vi "Auto Further Scale.vi"(10 "Time to wait (min 50ms)":dbl=100.0, 11 "Right?":bool=TRUE) -> ()   [LabVIEW 2017]
uses:
  LabVIEW_is_Under_Control.lib/Util/Unpack Gamepad/Button Cluster.ctl
  LabVIEW_is_Under_Control.lib/Util/Unpack Gamepad/D-Pad.ctl
  Team Code/Robot Global Data.vi
panel:
  out "Auto State":T1(ring)=enum."Finalizando"
  in  "Time_Limit_ Turn_2":dbl=1500.0 format="%#_13g"
  in  "Time_Limit_fwd_2":dbl=4500.0 format="%#_13g"
  in  "Time_Limit_Turn":dbl=2500.0 format="%#_13g"
  in  "Time_Limit_fwd":dbl=4000.0 format="%#_13g"
  in  "Time_Limit_fwd_3":dbl=2000.0 format="%#_13g"
  in  "Time to wait 3(min 50ms)":dbl=50.0
  in  "Delay Fwd 3":i32=100
  in  "DistanceScale":dbl=75.0
  in  "Delay Turn 2":i32=200
  in  "Turn 2":dbl=90.0 format="%#_13g"
  in  "Delay Fwd 2":i32=500
  in  "DistanceAfterTurn":dbl=450.0
  in  "Delay Turn":i32=600
  in  "Turn":dbl=-85.0 format="%#_13g"
  in  "Delay Fwd":i32=500
  in  "DistanceFwd":dbl=545.0
  in  "Time to wait 3 (min 50ms)":dbl=50.0
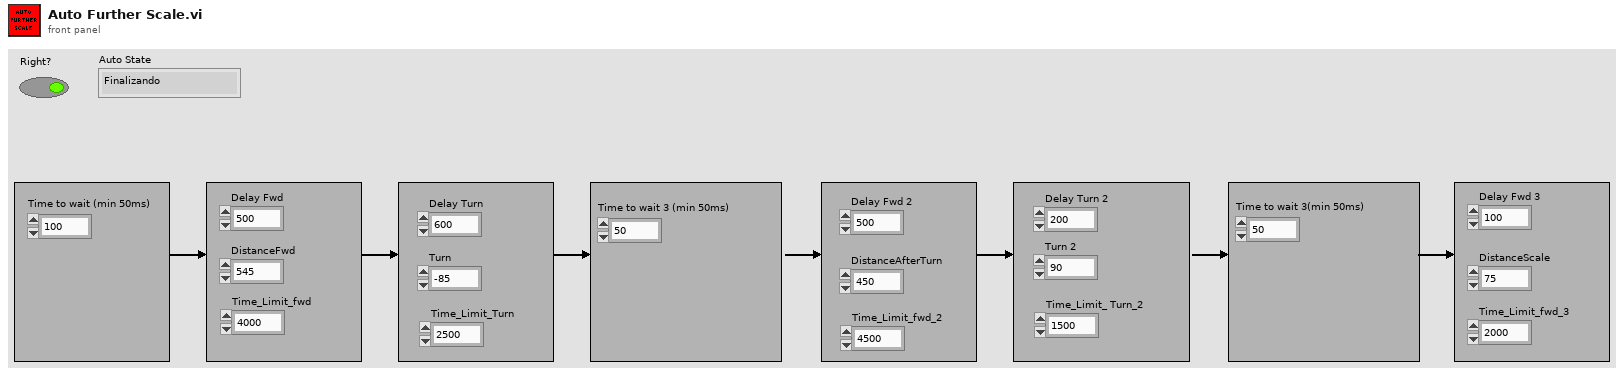
[diagram p1: front panel]
types:
  T1 = enum16{"Zerandosensor", "Andando", "Girando", "Zerandosensor2", "Andando2", "Girando2", "Zerandosensor3", "Andando3", "Score", "Finalizando", "Jogando"}
  T2 = enum16{"Zerandosensor", "Andando", "Girando", "Zerandosensor2", "Andando2", "Girando2", "Zerandosensor3", "Andando3", "Score", "Finalizando"}
  T3 = typedef "Button Cluster.ctl" = cluster{"Buttons[0]":bool, "Buttons[1]":bool, "Buttons[2]":bool, "Buttons[3]":bool, "Buttons[4]":bool, "Buttons[5]":bool, "Buttons[6]":bool, "Buttons[7]":bool, "Buttons[8]":bool, "Buttons[9]":bool}
  T4 = cluster{"proportional gain (Kc)":dbl, "integral time (Ti, min)":dbl, "derivative time (Td, min)":dbl}
  T5 = typedef "D-Pad.ctl" = cluster{"Top":bool, "Bottom":bool, "None":bool, "Right":bool, "Left":bool}
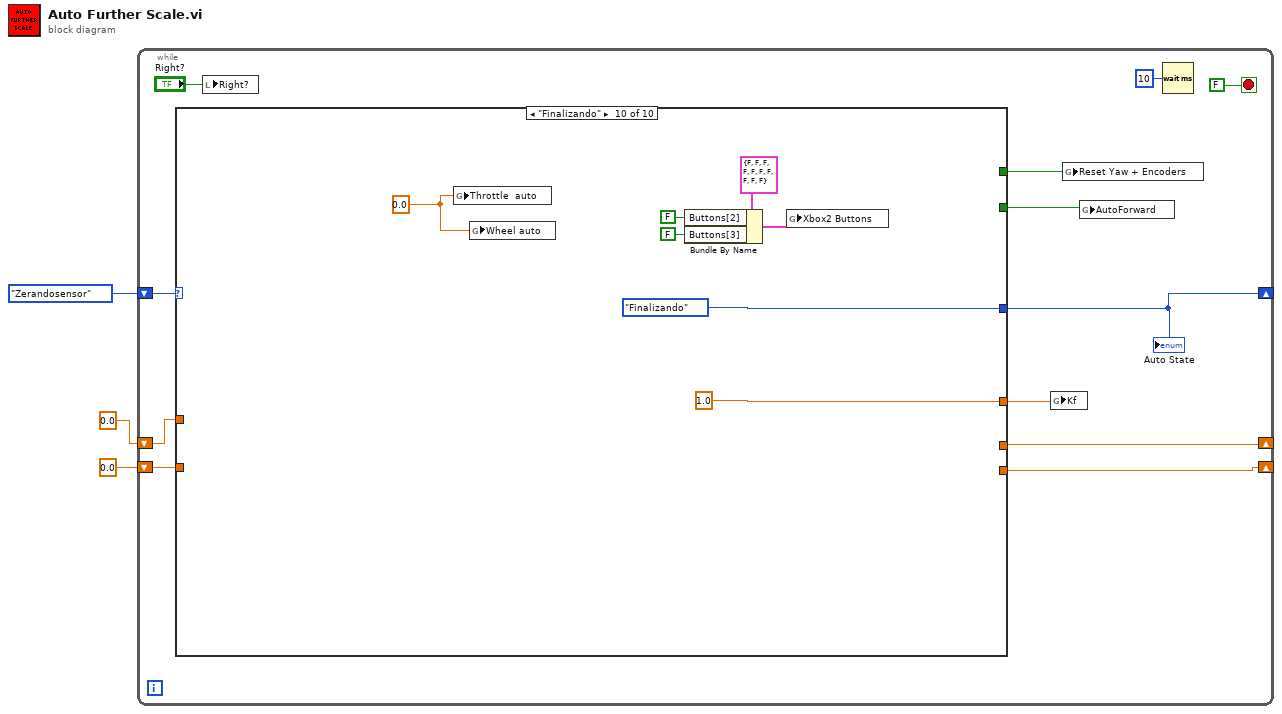
[diagram p0: block diagram]
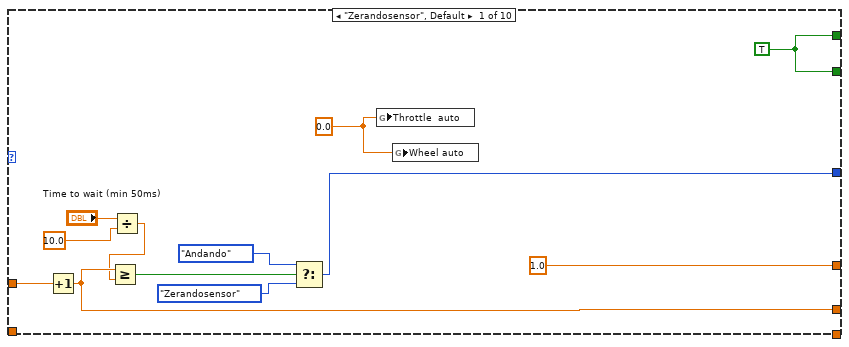
[diagram p2: hidden frame]
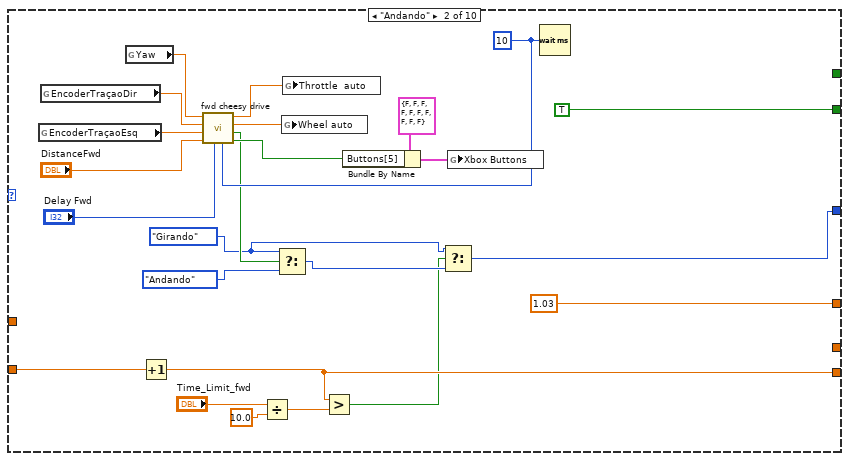
[diagram p3: hidden frame]
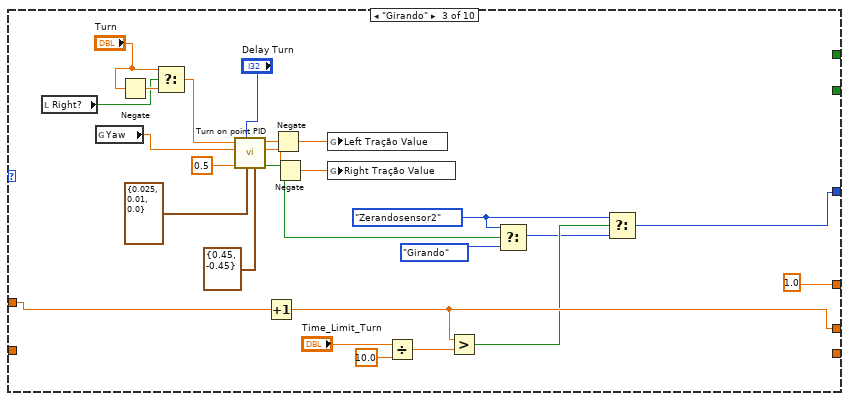
[diagram p4: hidden frame]
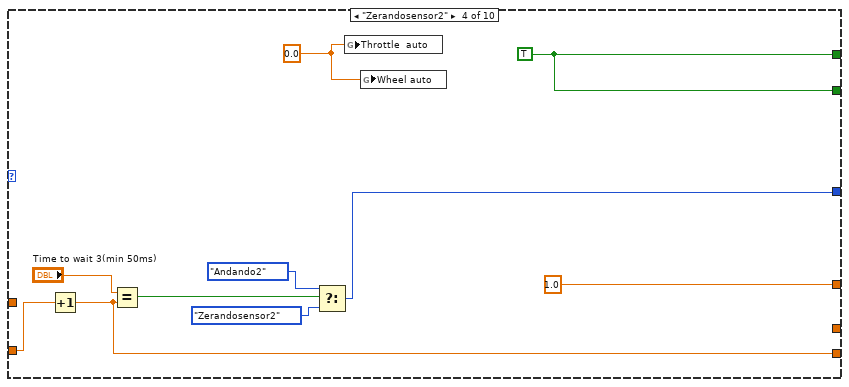
[diagram p5: hidden frame]
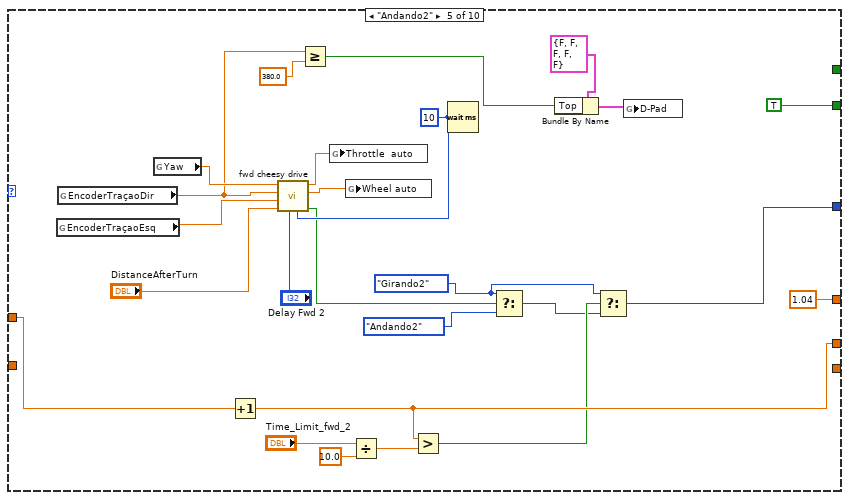
[diagram p6: hidden frame]
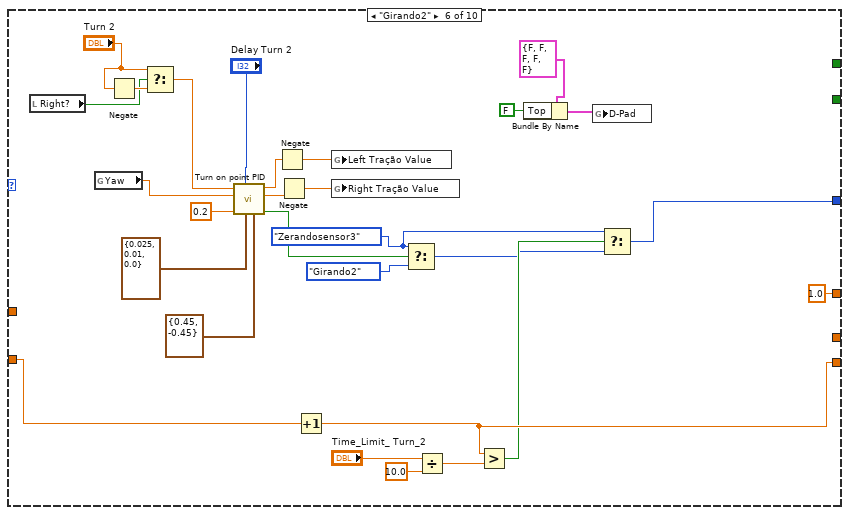
[diagram p7: hidden frame]
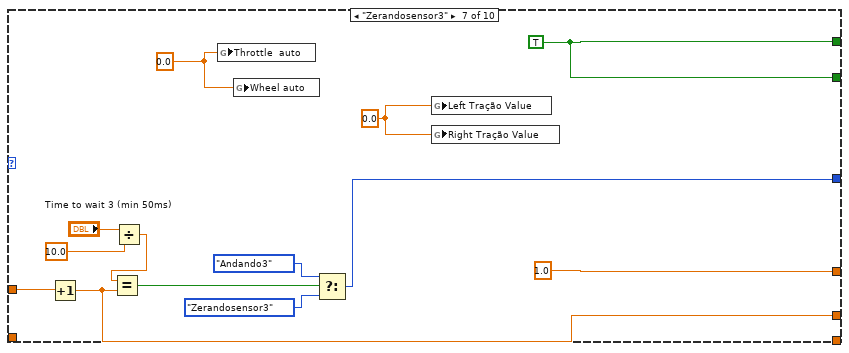
[diagram p8: hidden frame]
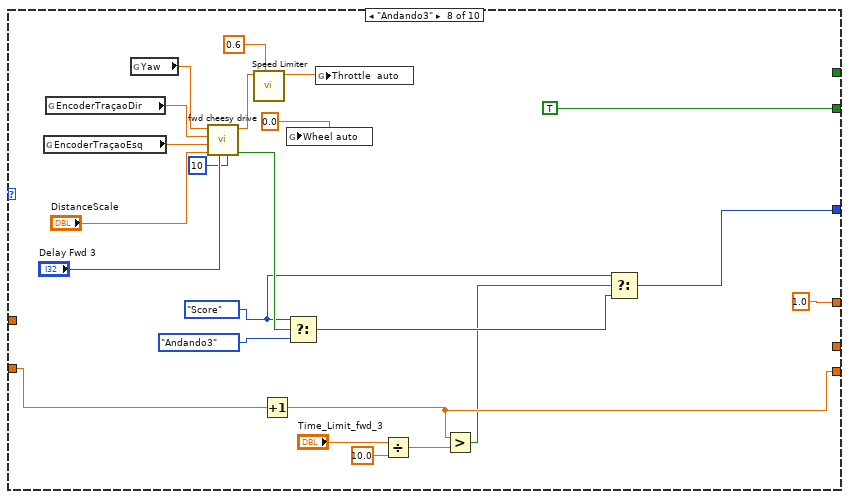
[diagram p9: hidden frame]
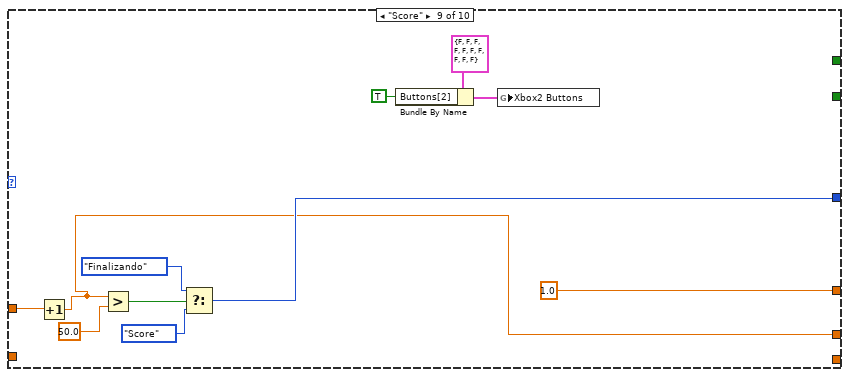
[diagram p10: hidden frame]
diagram:
  n1 = while {
    shift-right: [w7] -> _
    shift-left: T2."Zerandosensor" -> [w6]
    shift-right: [w9] -> _
    shift-left: 0.0 -> [w10]
    shift-right: [w4] -> _
    shift-left: 0.0 -> [w5]
    stop <- FALSE stop-if-true
    n2 = case shown="\"Finalizando\"" w6 {
      tunnel: [w27 _ _ w84 _ _ w144 _ _ _] -> w12
      tunnel: [w27 TRUE _ w84 TRUE _ w144 TRUE _ _] -> w13
      tunnel: [1.0 1.03 1.0 1.0 1.04 1.0 1.0 1.0 1.0 1.0] -> w11
      tunnel: w10 -> [w23 _ w57 _ w97 _ w149 _ w186 _]
      tunnel: [w17 _ w56 _ w96 _ w146 _ w179 _] -> w9
      tunnel: [w20 w32 w55 w82 w92 w119 w143 w162 w180 T1."Finalizando"] -> w7
      tunnel: w5 -> [_ w34 _ w78 _ w121 _ w164 _ _]
      tunnel: [_ w33 _ w77 _ w120 _ w163 _ _] -> w4
      frame "Zerandosensor", Default {
        w21 = 0.0
        w27 = TRUE
        n3 = Increment(x=w23) -> (x+1=w17:dbl)
        n4 = Divide(x="Time to wait (min 50ms)", y=10.0) -> (x/y=w16:dbl)
        n5 = Greater Or Equal?(x=w17, y=w16) -> (x >= y?=w22:bool)
        n6 = Select(t=T2."Andando", s=w22, f=T2."Zerandosensor") -> (s? t:f=w20:T2)
        n7 = global write "Robot Global Data.vi" "Throttle  auto"(w21) -> ()
        n8 = global write "Robot Global Data.vi" "Wheel auto"(w21) -> ()
      }
      frame "Andando" {
        w29 = T2."Girando"
        w45 = u32 10 ("milliseconds to wait")
        n9 = global read "Robot Global Data.vi" "EncoderTraçaoEsq"() -> (w48:dbl)
        n10 = global read "Robot Global Data.vi" "EncoderTraçaoDir"() -> (w47:dbl)
        n11 = global read "Robot Global Data.vi" "Yaw"() -> (w49:dbl)
        n12 = Increment(x=w34) -> (x+1=w33:dbl)
        n13 = call "fwd cheesy drive.vi"("Loop Timer"=w45, "Time to stop"="Delay Fwd", "Distance"="DistanceFwd", "Encoder Left"=w48, "Encoder Right"=w47, "Yaw"=w49) -> ("Finished distance"=w40:bool, "Both finished"=w39:bool, "Direction"=w44:dbl, "Trottle"=w43:dbl)  [unwired: 2 in]
        n14 = Divide(x="Time_Limit_fwd", y=10.0) -> (x/y=w37:dbl)
        n15 = Select(t=w29, s=w39, f=T2."Andando") -> (s? t:f=w30:T2)
        n16 = global write "Robot Global Data.vi" "Wheel auto"(w44) -> ()
        n17 = global write "Robot Global Data.vi" "Throttle  auto"(w43) -> ()
        n18 = Greater?(x=w33, y=w37) -> (0:w28:bool)
        n19 = Bundle By Name(cluster=T3 {"Buttons[0]"=FALSE, "Buttons[1]"=FALSE, "Buttons[2]"=FALSE, "Buttons[3]"=FALSE, "Buttons[4]"=FALSE, "Buttons[5]"=FALSE, "Buttons[6]"=FALSE, "Buttons[7]"=FALSE, "Buttons[8]"=FALSE, "Buttons[9]"=FALSE} ("Xbox Buttons"), "Buttons[5]"=w40) -> (w41:T3)
        n20 = Select(t=w29, s=w28, f=w30) -> (s? t:f=w32:T2)
        n21 = global write "Robot Global Data.vi" "Xbox Buttons"(w41) -> ()
        n22 = Wait (ms)(milliseconds to wait=w45) -> ()  [unwired: 1 out]
      }
      frame "Girando" {
        w52 = T2."Zerandosensor2"
        n23 = local read "Right?"() -> (w64:bool)
        n24 = global read "Robot Global Data.vi" "Yaw"() -> (w70:dbl)
        n25 = Negate(x="Turn") -> (-x=w67:dbl)
        n26 = Select(t="Turn", s=w64, f=w67) -> (s? t:f=w65:dbl)
        n27 = call "Turn on point PID.vi"("Range"=cluster{"output high":dbl, "output low":dbl} {"output high"=0.45, "output low"=-0.45}, "Gains"=T4 {"proportional gain (Kc)"=0.025, "integral time (Ti, min)"=0.01, "derivative time (Td, min)"=0.0}, "Time to stop"="Delay Turn", "Precision"=0.5, "Yaw"=w70, "Setpoint(degrees)"=w65) -> ("Finished?"=w74:bool, "PWM right"=w71:dbl, "PWM left"=w72:dbl)  [unwired: 3 in]
        n28 = Increment(x=w57) -> (x+1=w56:dbl)
        n29 = Negate(x=w72) -> (-x=w69:dbl)
        n30 = Negate(x=w71) -> (-x=w68:dbl)
        n31 = global write "Robot Global Data.vi" "Left Tração Value"(w69) -> ()
        n32 = global write "Robot Global Data.vi" "Right Tração Value"(w68) -> ()
        n33 = Divide(x="Time_Limit_Turn", y=10.0) -> (x/y=w59:dbl)
        n34 = Greater?(x=w56, y=w59) -> (0:w54:bool)
        n35 = Select(t=w52, s=w74, f=T2."Girando") -> (s? t:f=w53:T2)
        n36 = Select(t=w52, s=w54, f=w53) -> (s? t:f=w55:T2)
      }
      frame "Zerandosensor2" {
        w86 = 0.0
        w84 = TRUE
        n37 = Increment(x=w78) -> (x+1=w77:dbl)
        n38 = Equal?(x="Time to wait 3(min 50ms)", y=w77) -> (x = y?=w83:bool)
        n39 = Select(t=T2."Andando2", s=w83, f=T2."Zerandosensor2") -> (s? t:f=w82:T2)
        n40 = global write "Robot Global Data.vi" "Throttle  auto"(w86) -> ()
        n41 = global write "Robot Global Data.vi" "Wheel auto"(w86) -> ()
      }
      frame "Andando2" {
        w93 = T2."Girando2"
        w106 = u32 10 ("milliseconds to wait")
        n42 = global read "Robot Global Data.vi" "EncoderTraçaoEsq"() -> (w108:dbl)
        n43 = global read "Robot Global Data.vi" "EncoderTraçaoDir"() -> (w91:dbl)
        n44 = global read "Robot Global Data.vi" "Yaw"() -> (w109:dbl)
        n45 = Increment(x=w97) -> (x+1=w96:dbl)
        n46 = call "fwd cheesy drive.vi"("Loop Timer"=w106, "Time to stop"="Delay Fwd 2", "Distance"="DistanceAfterTurn", "Encoder Left"=w108, "Encoder Right"=w91, "Yaw"=w109) -> ("Finished distance"=w101:bool, "Direction"=w104:dbl, "Trottle"=w103:dbl)  [unwired: 2 in, 1 out]
        n47 = Greater Or Equal?(x=w91, y=380.0) -> (x >= y?=w87:bool)
        n48 = global write "Robot Global Data.vi" "Throttle  auto"(w103) -> ()
        n49 = global write "Robot Global Data.vi" "Wheel auto"(w104) -> ()
        n50 = Divide(x="Time_Limit_fwd_2", y=10.0) -> (x/y=w99:dbl)
        n51 = Greater?(x=w96, y=w99) -> (0:w95:bool)
        n52 = Wait (ms)(milliseconds to wait=w106) -> ()  [unwired: 1 out]
        n53 = Select(t=w93, s=w101, f=T2."Andando2") -> (s? t:f=w94:T2)
        n54 = Bundle By Name(cluster=T5 {"Top"=FALSE, "Bottom"=FALSE, "None"=FALSE, "Right"=FALSE, "Left"=FALSE} ("D-Pad"), "Top"=w87) -> (w89:T5)
        n55 = Select(t=w93, s=w95, f=w94) -> (s? t:f=w92:T2)
        n56 = global write "Robot Global Data.vi" "D-Pad"(w89) -> ()
      }
      frame "Girando2" {
        w118 = T2."Zerandosensor3"
        n57 = local read "Right?"() -> (w127:bool)
        n58 = global read "Robot Global Data.vi" "Yaw"() -> (w133:dbl)
        n59 = Negate(x="Turn 2") -> (-x=w130:dbl)
        n60 = Select(t="Turn 2", s=w127, f=w130) -> (s? t:f=w128:dbl)
        n61 = call "Turn on point PID.vi"("Range"=cluster{"output high":dbl, "output low":dbl} {"output high"=0.45, "output low"=-0.45}, "Gains"=T4 {"proportional gain (Kc)"=0.025, "integral time (Ti, min)"=0.01, "derivative time (Td, min)"=0.0}, "Time to stop"="Delay Turn 2", "Precision"=0.2, "Yaw"=w133, "Setpoint(degrees)"=w128) -> ("Finished?"=w137:bool, "PWM right"=w134:dbl, "PWM left"=w135:dbl)  [unwired: 3 in]
        n62 = Negate(x=w135) -> (-x=w132:dbl)
        n63 = Negate(x=w134) -> (-x=w131:dbl)
        n64 = Increment(x=w121) -> (x+1=w120:dbl)
        n65 = global write "Robot Global Data.vi" "Left Tração Value"(w132) -> ()
        n66 = global write "Robot Global Data.vi" "Right Tração Value"(w131) -> ()
        n67 = Select(t=w118, s=w137, f=T2."Girando2") -> (s? t:f=w115:T2)
        n68 = Divide(x="Time_Limit_ Turn_2", y=10.0) -> (x/y=w123:dbl)
        n69 = Greater?(x=w120, y=w123) -> (0:w116:bool)
        n70 = Bundle By Name(cluster=T5 {"Top"=FALSE, "Bottom"=FALSE, "None"=FALSE, "Right"=FALSE, "Left"=FALSE} ("D-Pad"), "Top"=FALSE) -> (w114:T5)
        n71 = global write "Robot Global Data.vi" "D-Pad"(w114) -> ()
        n72 = Select(t=w118, s=w116, f=w115) -> (s? t:f=w119:T2)
      }
      frame "Zerandosensor3" {
        w140 = 0.0
        w144 = TRUE
        w147 = 0.0
        n73 = Increment(x=w149) -> (x+1=w146:dbl)
        n74 = Divide(x="Time to wait 3 (min 50ms)", y=10.0) -> (x/y=w150:dbl)
        n75 = Equal?(x=w150, y=w146) -> (x = y?=w148:bool)
        n76 = global write "Robot Global Data.vi" "Throttle  auto"(w147) -> ()
        n77 = global write "Robot Global Data.vi" "Wheel auto"(w147) -> ()
        n78 = Select(t=T2."Andando3", s=w148, f=T2."Zerandosensor3") -> (s? t:f=w143:T2)
        n79 = global write "Robot Global Data.vi" "Left Tração Value"(w140) -> ()
        n80 = global write "Robot Global Data.vi" "Right Tração Value"(w140) -> ()
      }
      frame "Andando3" {
        w160 = T2."Score"
        n81 = global read "Robot Global Data.vi" "EncoderTraçaoEsq"() -> (w172:dbl)
        n82 = global read "Robot Global Data.vi" "EncoderTraçaoDir"() -> (w171:dbl)
        n83 = global read "Robot Global Data.vi" "Yaw"() -> (w173:dbl)
        n84 = call "fwd cheesy drive.vi"("Loop Timer"=10, "Time to stop"="Delay Fwd 3", "Distance"="DistanceScale", "Encoder Left"=w172, "Encoder Right"=w171, "Yaw"=w173) -> ("Finished distance"=w168:bool, "Trottle"=w154:dbl)  [unwired: 2 in, 2 out]
        n85 = call "Speed Limiter.vi"("Limit"=0.6, "Motor Input"=w154) -> ("Output"=w155:dbl)  [unwired: 9 in]
        n86 = Increment(x=w164) -> (x+1=w163:dbl)
        n87 = global write "Robot Global Data.vi" "Wheel auto"(0.0 ("Wheel auto")) -> ()
        n88 = Select(t=w160, s=w168, f=T2."Andando3") -> (s? t:f=w159:T2)
        n89 = global write "Robot Global Data.vi" "Throttle  auto"(w155) -> ()
        n90 = Divide(x="Time_Limit_fwd_3", y=10.0) -> (x/y=w167:dbl)
        n91 = Greater?(x=w163, y=w167) -> (0:w158:bool)
        n92 = Select(t=w160, s=w158, f=w159) -> (s? t:f=w162:T2)
      }
      frame "Score" {
        n93 = Increment(x=w186) -> (x+1=w179:dbl)
        n94 = Greater?(x=w179, y=50.0) -> (0:w184:bool)
        n95 = Select(t=T1."Finalizando", s=w184, f=T1."Score") -> (s? t:f=w180:T1)
        n96 = Bundle By Name(cluster=T3 {"Buttons[0]"=FALSE, "Buttons[1]"=FALSE, "Buttons[2]"=FALSE, "Buttons[3]"=FALSE, "Buttons[4]"=FALSE, "Buttons[5]"=FALSE, "Buttons[6]"=FALSE, "Buttons[7]"=FALSE, "Buttons[8]"=FALSE, "Buttons[9]"=FALSE} ("Xbox Buttons"), "Buttons[2]"=TRUE) -> (w177:T3)
        n97 = global write "Robot Global Data.vi" "Xbox2 Buttons"(w177) -> ()
      }
      frame "Finalizando" {
        w193 = 0.0
        n98 = global write "Robot Global Data.vi" "Throttle  auto"(w193) -> ()
        n99 = global write "Robot Global Data.vi" "Wheel auto"(w193) -> ()
        n100 = Bundle By Name(cluster=T3 {"Buttons[0]"=FALSE, "Buttons[1]"=FALSE, "Buttons[2]"=FALSE, "Buttons[3]"=FALSE, "Buttons[4]"=FALSE, "Buttons[5]"=FALSE, "Buttons[6]"=FALSE, "Buttons[7]"=FALSE, "Buttons[8]"=FALSE, "Buttons[9]"=FALSE} ("Xbox Buttons"), "Buttons[2]"=FALSE, "Buttons[3]"=FALSE) -> (w189:T3)
        n101 = global write "Robot Global Data.vi" "Xbox2 Buttons"(w189) -> ()
      }
    }
    "Auto State" <- w7
    n102 = local write "Right?"("Right?") -> ()
    n103 = global write "Robot Global Data.vi" "Kf"(w11) -> ()
    n104 = global write "Robot Global Data.vi" "Reset Yaw + Encoders"(w12) -> ()
    n105 = global write "Robot Global Data.vi" "AutoForward"(w13) -> ()
    n106 = Wait (ms)(milliseconds to wait=u32 10) -> ()  [unwired: 1 out]
  }
